vi "calibrate polarizer.vi"() -> ()   [LabVIEW 2018, in "Power Meter.lvlib"]
uses:
  Power Meter.lvlib
  Laser/Laser.lvlib
  C:/FlashGordon/Development/dll/ThorLabs.MotionControl.KCube.DCServoCLI.dll
  dll/ThorLabs.MotionControl.KCube.DCServoCLI.dll
panel:
  out "Angles":dbl[](array[numeric])
  out "Angle":dbl
  out "Power":dbl
  in  "error in (no error)":errorcluster {"code" format="%.0x"}
  out "Power":dbl[](array[numeric])
  in  "Stop Button":bool
  out "error out":errorcluster
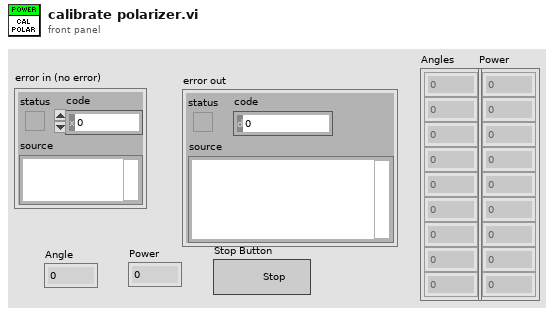
[diagram p1: front panel]
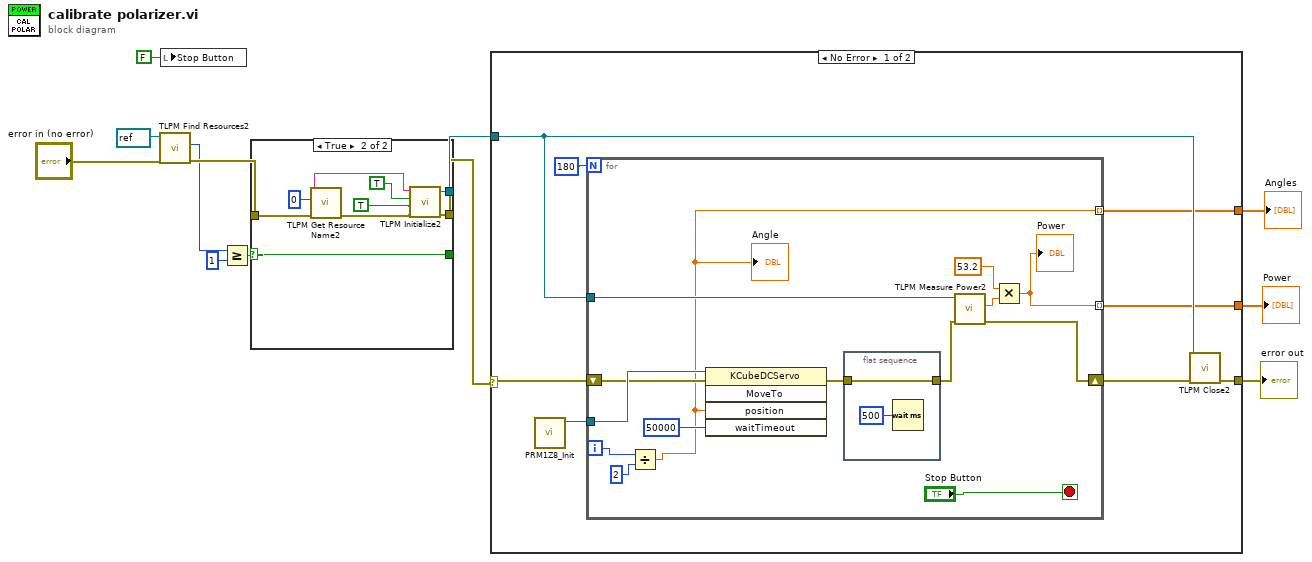
[diagram p0: block diagram]
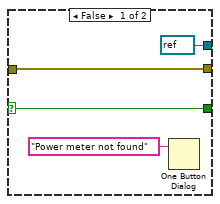
[diagram p3: hidden frame]
diagram:
  n1 = call "TLPM Find Resources2.vi"("error in (no error)"="error in (no error)", "instrument handle"=refnum<visa-resource-name> refnum) -> ("error out"=w6:errorcluster, "Resource Count"=w5:u32)  [unwired: 7 in, 1 out]
  n2 = local write "Stop Button"(FALSE ("Stop Button")) -> ()
  n3 = Greater Or Equal?(x=w5, y=u32 1) -> (x >= y?=w7:bool)
  n4 = case shown="True" w7 {
    selector: w7 -> [w15 w25]
    tunnel: [refnum<visa-resource-name> refnum ("instrument handle out") w20] -> w12
    tunnel: w6 -> [w14 w24]
    tunnel: [w15 w25] -> _
    tunnel: [w14 w21] -> w2
    frame False {
      n5 = One Button Dialog(message="Power meter not found") -> ()  [unwired: 1 in, 1 out]
    }
    frame True {
      n6 = call "TLPM Get Resource Name2.vi"("error in (no error)"=w24, "Index (0)"=u32 0 ("Device Index")) -> ("error out"=w22:errorcluster, "Resource Name"=w17:string)  [unwired: 7 in, 1 out]
      n7 = call "TLPM Initialize2.vi"("error in (no error)"=w22, "Reset Device (Reset Device)"=TRUE ("ID Query (Do Query)"), "ID Query (Do Query)"=TRUE, "resource name"=w17) -> ("error out"=w21:errorcluster, "instrument handle out"=w20:refnum<visa-resource-name>)  [unwired: 6 in]
    }
  }
  n8 = case shown="No Error" w2 {
    selector: w2 -> [w27 w50]
    tunnel: w12 -> [w33 _]
    tunnel: [w30 _] -> w11
    tunnel: [w28 w50] -> w10
    tunnel: [w26 _] -> w1
    frame No Error {
      n9 = call "PRM1Z8_Init.vi"() -> ("reference out"=w32:refnum<k24>)  [unwired: 10 in, 1 out]
      n10 = for {
        N: 180 -> [_]
        tunnel: w33 -> [w47]
        tunnel: [w36] -> w30 mode=indexing
        tunnel: w32 -> [w45]
        shift-right: [w44] -> w29
        shift-left: w27 -> [w43]
        tunnel: [w34] -> w26 mode=indexing
        i -> [w39]
        stop <- "Stop Button" stop-if-true
        n11 = Divide(x=w39, y=2) -> (x/y=w34:dbl)
        "Angle" <- w34
        n12 = invoke class="KCubeDCServo" method="MoveTo"(reference=w45, error in=w43, "position"=w34, "waitTimeout"=50000) -> (error out=w41:errorcluster)  [unwired: 1 in, 4 out]
        n13 = flat-sequence {
          tunnel: w41 -> [w49]
          tunnel: [w49] -> w40
          frame #0 {
            n14 = Wait (ms)(milliseconds to wait=u32 500) -> ()  [unwired: 1 out]
          }
        }
        n15 = call "TLPM Measure Power2.vi"("error in (no error)"=w40, "instrument handle"=w47) -> ("error out"=w44:errorcluster, "Power"=w37:dbl)  [unwired: 7 in, 1 out]
        n16 = Multiply(x=53.2, y=w37) -> (x*y=w36:dbl)
        "Power" <- w36
      }
      n17 = call "TLPM Close2.vi"("error in (no error)"=w29, "instrument handle"=w33) -> ("error out"=w28:errorcluster)  [unwired: 9 in]
    }
    frame Error {
    }
  }
  "error out" <- w10
  "Power" <- w11
  "Angles" <- w1
